vi "array reverse.vi"() -> ()   [LabVIEW 2015]
panel:
  out "Array 2":dbl[](array[numeric])
  out "Array":dbl[](array[numeric])
  in  "Enter array index":dbl
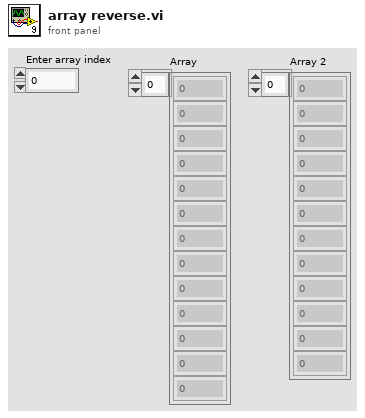
[diagram p1: front panel]
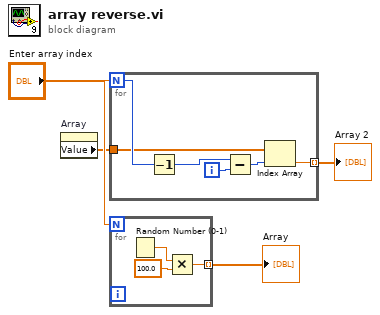
[diagram p0: block diagram]
diagram:
  n1 = property on="Array" class="Arr (strict)"() -> ("Value"=w2:dbl[])  [unwired: 2 in, 2 out]
  n2 = for {
    N: "Enter array index" -> [w10]
    tunnel: w2 -> [w7]
    tunnel: [w5] -> w1 mode=indexing
    i -> [w6]
    n3 = Decrement(x=w10) -> (x-1=w9:i32)
    n4 = Subtract(x=w9, y=w6) -> (x-y=w8:i32)
    n5 = Index Array(array=w7, index=w8) -> (element=w5:dbl)
  }
  "Array 2" <- w1
  n6 = for {
    N: "Enter array index" -> [_]
    tunnel: [w11] -> w4 mode=indexing
    n7 = Random Number (0-1)() -> (number: 0 to 1=w13:dbl)
    n8 = Multiply(x=w13, y=100.0) -> (x*y=w11:dbl)
  }
  "Array" <- w4
